vi "laserOnOff.vi"(8 "error in (no error)":errorcluster, 9 "Emission (F = OFF)":bool, 10 "Power, mW (100)":dbl=100.0, 11 "VISA Refnum in":refnum<visa-resource-name>) -> (0 "error out":errorcluster, 2 "Power, mW":dbl, 3 "VISA Refnum out":refnum<visa-resource-name>)   [LabVIEW 2011]
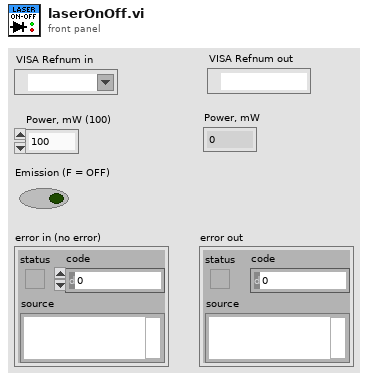
[diagram p1: front panel]
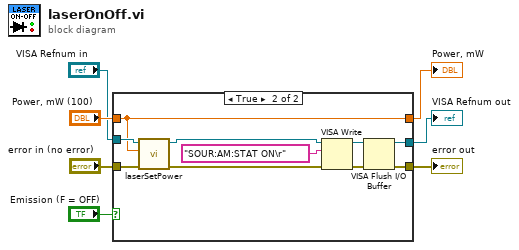
[diagram p0: block diagram]
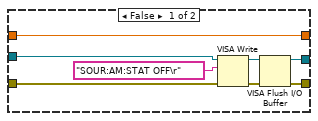
[diagram p2: hidden frame]
diagram:
  n1 = case shown="True" "Emission (F = OFF)" {
    tunnel: "error in (no error)" -> [w11 w20]
    tunnel: "VISA Refnum in" -> [w14 w19]
    tunnel: [w9 w22] -> w5
    tunnel: [w12 w21] -> w1
    tunnel: "Power, mW (100)" -> [w15 w16]
    tunnel: [w15 w16] -> w2
    frame False {
      n2 = VISA Write(VISA resource name=w14, write buffer="SOUR:AM:STAT OFF\r", error in (no error)=w11) -> (VISA resource name out=w13:refnum<visa-resource-name>, error out=w10:errorcluster)  [unwired: 1 out]
      n3 = VISA Flush I/O Buffer(VISA resource name=w13, error in (no error)=w10) -> (VISA resource name out=w12:refnum<visa-resource-name>, error out=w9:errorcluster)  [unwired: 1 in]
    }
    frame True {
      n4 = call "laserSetPower.vi"("error in (no error)"=w20, "Laser Power (mW)"=w16, "VISA Refnum in"=w19) -> ("error out"=w17:errorcluster, "VISA Refnum out"=w18:refnum<visa-resource-name>)  [unwired: 7 in]
      n5 = VISA Write(VISA resource name=w18, write buffer="SOUR:AM:STAT ON\r", error in (no error)=w17) -> (VISA resource name out=w24:refnum<visa-resource-name>, error out=w25:errorcluster)  [unwired: 1 out]
      n6 = VISA Flush I/O Buffer(VISA resource name=w24, error in (no error)=w25) -> (VISA resource name out=w21:refnum<visa-resource-name>, error out=w22:errorcluster)  [unwired: 1 in]
    }
  }
  "error out" <- w5
  "Power, mW" <- w2
  "VISA Refnum out" <- w1
